vi "Constructor Singleton.vi"(6 "Enum":enum16{"Init", "Update"}(ring), 11 "Excel Logger.lvclass 2":refnum<class "Excel Logger.lvclass">) -> (3 "Excel Logger.lvclass":refnum<class "Excel Logger.lvclass">)   [LabVIEW 2016, in "Excel Logger.lvclass"]
uses:
  Excel Logger.lvclass
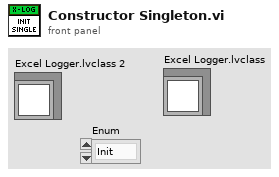
[diagram p1: front panel]
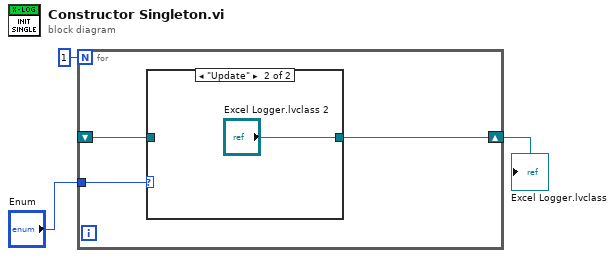
[diagram p0: block diagram]
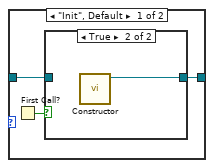
[diagram p2: hidden frame]
diagram:
  n1 = for {
    N: 1 -> [_]
    shift-right: [w5] -> w2
    shift-left: _ -> [w6]
    tunnel: "Enum" -> [w4]
    n2 = case shown="\"Update\"" w4 {
      tunnel: w6 -> [w9 _]
      tunnel: [w7 "Excel Logger.lvclass 2"] -> w5
      frame "Init", Default {
        n3 = First Call?() -> (First Call?: T/F=w8:bool)
        n4 = case shown="True" w8 {
          tunnel: w9 -> [w10 _]
          tunnel: [w10 w11] -> w7
          frame False {
          }
          frame True {
            n5 = call "Constructor.vi"() -> ("Excel Logger.lvclass"=w11:refnum<class "Excel Logger.lvclass">)  [unwired: 11 in]
          }
        }
      }
      frame "Update" {
      }
    }
  }
  "Excel Logger.lvclass" <- w2
